vi "3458A Initiate Digitizing Process.vi"(8 "error in":errorcluster, 9 "Is first multiplex cycle? (True)":bool, 11 "session in":T1={"channels"=[], "sync unit"={"VISA"="", "type"=enum."Picotest U6200A"}, "awg unit"={"type"=enum."Agilent 331xxA to 332xxA", "VISA"="", "enable 10MHz ref"=FALSE, "cmi ckd2"={"VISA"="", "clock source"=enum."Auto", "manual ref clk"=FALSE, "ref clock [Hz]"=0.0, "div mode"=enum."Set divisor directly"}, "cmi sync v3"={"VISA"="", "baud rate [bd/s]"=115200, "source"=enum."Auto", "hv range"=enum."1kV", "fsrc is fixed"=FALSE, "fsrc [Hz]"=10000000.0, "freq integ [s]"=1.0, "freq filter"=5, "trig level"=enum."TTL 5V", "chn1 mode"=enum."Source divider", "chn1 level"=enum."Positive 5V", "chn2 mode"=enum."Source divider", "chn2 level"=enum."Positive 5V", "chn2 div"=1, "chn3 mode"=enum."Chn 1 Active", "chn3 level"=enum."Positive 5V", "chn1 div entry"=enum."Calculate nearest divisor from measured fx", "chn1 dev limit [%]"=1.0, "chn1 check dev"=FALSE}, "trigger"={"source"=enum."Immediate", "slope"=enum."POS", "coupling"=enum."DC", "level [V]"=0.0, "hysteresis [V]"=0.0, "pre-trigger [%]"=0.0}, "HMF2500 cfg"={"Baud Rate"=9600, "Parity"=0, "Data Bits"=8, "Flow Control"=4}}, "sync mode"=enum."MASTER-SLAVE, MASTER clocked by TIMER", "streaming mode"=FALSE, "idn mode"=enum."Auto", "sampling mode"=enum."DCV", "sample memory [B]"=0, "proc setup"={"channel id"=0, "packet size [smpl]"=0, "current timeout [s]"=0.0, "blk2blk timeout [s]"=0.0, "event time"=timestamp(0 s since 1904-01-01), "stop notifier"=refnum, "data queues"=[], "proc refs"=[], "bus semaphore"=refnum}, "sample size [B]"=0, "sample count"=0, "aux data"={"channel id"=0, "valid?"=[], "gain [V]"=[], "timestamp [s]"=[], "Ts [s]"=0.0, "abs timestamp"=timestamp(0 s since 1904-01-01), "t [deg C]"=[], "multiplex timestamp [s]"=-1.0, "only multiplex?"=FALSE, "multiplex smpl offset"=0, "overflow?"=FALSE}, "ranges [V]"=[], "aperture [s]"=0.0, "LEVEL trigger"={"edge"=enum."POS", "level [V]"=0.0, "coupling"=enum."DC"}, "trigger mode"=enum."AUTO", "measure temp.?"=FALSE, "disp mesages"=[], "shared bus?"=FALSE, "disable display?"=FALSE, "aper mode"=enum."Manual", "aper rules"=[], "multiplex"={"cycles"=0, "delay [s]"=0.0, "enabled"=FALSE, "overhead [s]"=1.0, "tot smpls"=0, "sub-rec"=0, "overhead [%]"=0.0, "emulated"=FALSE}, "F8588 lpf"=enum."Off", "F8588 pll"=enum."Off", "F8588 couple"=enum."DC, auto", "fs"={"freq mode"=enum."fs or Ts", "fs [Hz]"=0.0, "fref [Hz]"=0.0, "mul"=0.0, "div"=0.0}, "fs mode"=enum."fs or Ts", "init timestamp"=timestamp(0 s since 1904-01-01), "last report timestamp"=timestamp(0 s since 1904-01-01)} {"awg unit"."HMF2500 cfg"."Flow Control" items=["None", "XON/XOFF", "RTS/CTS", "XON/XOFF & RTS/CTS", "DTR/DSR", "XON/XOFF & DTR/DSR"]; "awg unit"."HMF2500 cfg"."Data Bits" items=["7"=7, "8"=8]; "awg unit"."HMF2500 cfg"."Parity" items=["None", "Odd", "Even", "Mark", "Space"]; "awg unit"."HMF2500 cfg"."Baud Rate" items=["300"=300, "600"=600, "1200"=1200, "2400"=2400, "4800"=4800, "9600"=9600, "19200"=19200]; "awg unit"."cmi sync v3"."chn2 div" min=1 max=100000000 step=1; "awg unit"."cmi sync v3"."fsrc [Hz]" format="%_8p"; "channels"."Range [Vpk]" min=0.0}) -> (0 "error out":errorcluster, 2 "initiation timestamp":timestamp, 3 "session out":T1={"channels"=[], "sync unit"={"VISA"="", "type"=enum."Picotest U6200A"}, "awg unit"={"type"=enum."Agilent 331xxA to 332xxA", "VISA"="", "enable 10MHz ref"=FALSE, "cmi ckd2"={"VISA"="", "clock source"=enum."Auto", "manual ref clk"=FALSE, "ref clock [Hz]"=0.0, "div mode"=enum."Set divisor directly"}, "cmi sync v3"={"VISA"="", "baud rate [bd/s]"=115200, "source"=enum."Auto", "hv range"=enum."1kV", "fsrc is fixed"=FALSE, "fsrc [Hz]"=10000000.0, "freq integ [s]"=1.0, "freq filter"=5, "trig level"=enum."TTL 5V", "chn1 mode"=enum."Source divider", "chn1 level"=enum."Positive 5V", "chn2 mode"=enum."Source divider", "chn2 level"=enum."Positive 5V", "chn2 div"=1, "chn3 mode"=enum."Chn 1 Active", "chn3 level"=enum."Positive 5V", "chn1 div entry"=enum."Calculate nearest divisor from measured fx", "chn1 dev limit [%]"=1.0, "chn1 check dev"=FALSE}, "trigger"={"source"=enum."Immediate", "slope"=enum."POS", "coupling"=enum."DC", "level [V]"=0.0, "hysteresis [V]"=0.0, "pre-trigger [%]"=0.0}, "HMF2500 cfg"={"Baud Rate"=9600, "Parity"=0, "Data Bits"=8, "Flow Control"=4}}, "sync mode"=enum."MASTER-SLAVE, MASTER clocked by TIMER", "streaming mode"=FALSE, "idn mode"=enum."Auto", "sampling mode"=enum."DCV", "sample memory [B]"=0, "proc setup"={"channel id"=0, "packet size [smpl]"=0, "current timeout [s]"=0.0, "blk2blk timeout [s]"=0.0, "event time"=timestamp(0 s since 1904-01-01), "stop notifier"=refnum, "data queues"=[], "proc refs"=[], "bus semaphore"=refnum}, "sample size [B]"=0, "sample count"=0, "aux data"={"channel id"=0, "valid?"=[], "gain [V]"=[], "timestamp [s]"=[], "Ts [s]"=0.0, "abs timestamp"=timestamp(0 s since 1904-01-01), "t [deg C]"=[], "multiplex timestamp [s]"=-1.0, "only multiplex?"=FALSE, "multiplex smpl offset"=0, "overflow?"=FALSE}, "ranges [V]"=[], "aperture [s]"=0.0, "LEVEL trigger"={"edge"=enum."POS", "level [V]"=0.0, "coupling"=enum."DC"}, "trigger mode"=enum."AUTO", "measure temp.?"=FALSE, "disp mesages"=[], "shared bus?"=FALSE, "disable display?"=FALSE, "aper mode"=enum."Manual", "aper rules"=[], "multiplex"={"cycles"=0, "delay [s]"=0.0, "enabled"=FALSE, "overhead [s]"=1.0, "tot smpls"=0, "sub-rec"=0, "overhead [%]"=0.0, "emulated"=FALSE}, "F8588 lpf"=enum."Off", "F8588 pll"=enum."Off", "F8588 couple"=enum."DC, auto", "fs"={"freq mode"=enum."fs or Ts", "fs [Hz]"=0.0, "fref [Hz]"=0.0, "mul"=0.0, "div"=0.0}, "fs mode"=enum."fs or Ts", "init timestamp"=timestamp(0 s since 1904-01-01), "last report timestamp"=timestamp(0 s since 1904-01-01)} {"awg unit"."HMF2500 cfg"."Flow Control" items=["None", "XON/XOFF", "RTS/CTS", "XON/XOFF & RTS/CTS", "DTR/DSR", "XON/XOFF & DTR/DSR"]; "awg unit"."HMF2500 cfg"."Data Bits" items=["7"=7, "8"=8]; "awg unit"."HMF2500 cfg"."Parity" items=["None", "Odd", "Even", "Mark", "Space"]; "awg unit"."HMF2500 cfg"."Baud Rate" items=["300"=300, "600"=600, "1200"=1200, "2400"=2400, "4800"=4800, "9600"=9600, "19200"=19200]; "awg unit"."cmi sync v3"."chn2 div" min=1 max=100000000 step=1; "awg unit"."cmi sync v3"."fsrc [Hz]" format="%_8p"; "channels"."Range [Vpk]" min=0.0})   [LabVIEW 2020, in "3458A Virtual Digitizer.lvlib"]
doc: "Initiates acquisition for both single shot and streaming modes. It creates data queues and starts digitizing processes, one for each channel. If succeds the process immediatelly starts digitizing (after trigger event occures) and starts filling the queues with data. So this VI must be immediatelly followed by fetch loop that takes out data from the queue! This may be called repeatedely without calling 'Setup' function if multiple records are required with identical configuration.\n\nFor time multiplexing mode set 'Time multiplex mode = True'. When 'Is first multiplex cycle = True', it will initiate record of maximum possible size. For next multiplexing cycles set 'Is first multiplex cycle = False' which will just record timestamp. The timestamps from particular calls of this VI will be later used to split the long record to particular multiplexing sequence chunks."
uses:
  3458A Virtual Digitizer.lvlib
  3458A Digitizer Session.ctl
  3458A Virtual Channel Config.ctl
  Counter/Counter Session.ctl
  Counter/Counter Type.ctl
  AWG/AWG Session.ctl
  AWG/AWG Type.ctl
  AWG/CMI Clock Divider v2/CMI ckd2 Session.ctl
  AWG/CMI Clock Divider v2/CMI ckd2 Source Mode.ctl
  AWG/CMI Clock Divider v2/CMI ckd2 Divisor Mode.ctl
  AWG/CMI Sync V3/CMI Sync V3 session.ctl
  AWG/CMI Sync V3/Configure/CMI Sync V3 Reference Clock Source.ctl
  AWG/CMI Sync V3/Configure/CMI Sync V3 HV input Range.ctl
  AWG/CMI Sync V3/Configure/CMI Sync V3 Trigger Input Level.ctl
  AWG/CMI Sync V3/Configure/CMI Sync V3 Channel 1 Mode.ctl
  AWG/CMI Sync V3/Configure/CMI Sync V3 Channel Output Levels.ctl
  AWG/CMI Sync V3/Configure/CMI Sync V3 Channel 2 Mode.ctl
  AWG/CMI Sync V3/Configure/CMI Sync V3 Channel 3 Mode.ctl
  AWG/CMI Sync V3/Configure/CMI Sync V3 Channel 1 Divisor Entry Mode.ctl
  adc/ADC Trig Config.ctl
  adc/ADC Trig Mode Source.ctl
  adc/ADC Trig Slope.ctl
  adc/ADC Trig Coupling.ctl
  AWG/RaS HMF2500/HMF2500 Config.ctl
  3458A Sync Mode.ctl
  3458A Idn Mode.ctl
  3458A Digitizing Low Levels/Configure/Sampling Mode.ctl
  3458A Digitizing Process Options.ctl
  3458A Data Packet.ctl
  3458A Aux Record Data.ctl
  3458A Digitizing Low Levels/Configure/Level Setup.ctl
  3458A Digitizing Low Levels/Configure/First Sample Trigger.ctl
  3458A Aperture Selection Mode.ctl
  3458A Multiplexing Config.ctl
  Fluke 8588A/F8588A Low Pass Filter.ctl
  Fluke 8588A/F8588A Phase Lock.ctl
  Fluke 8588A/F8588A Coupling.ctl
  3458A Sampling Rate.ctl
  AWG/AWG Clock Setup Mode.ctl
  3458A Sample Rate Mode.ctl
  AWG/AWG.lvlib
  Counter/Counter.lvlib
  3458A Digitizing Low Levels/3458A Digitizing Low Levels.lvlib
  AWG/CMI Sync V3/CMI Sync Unit V3.lvlib
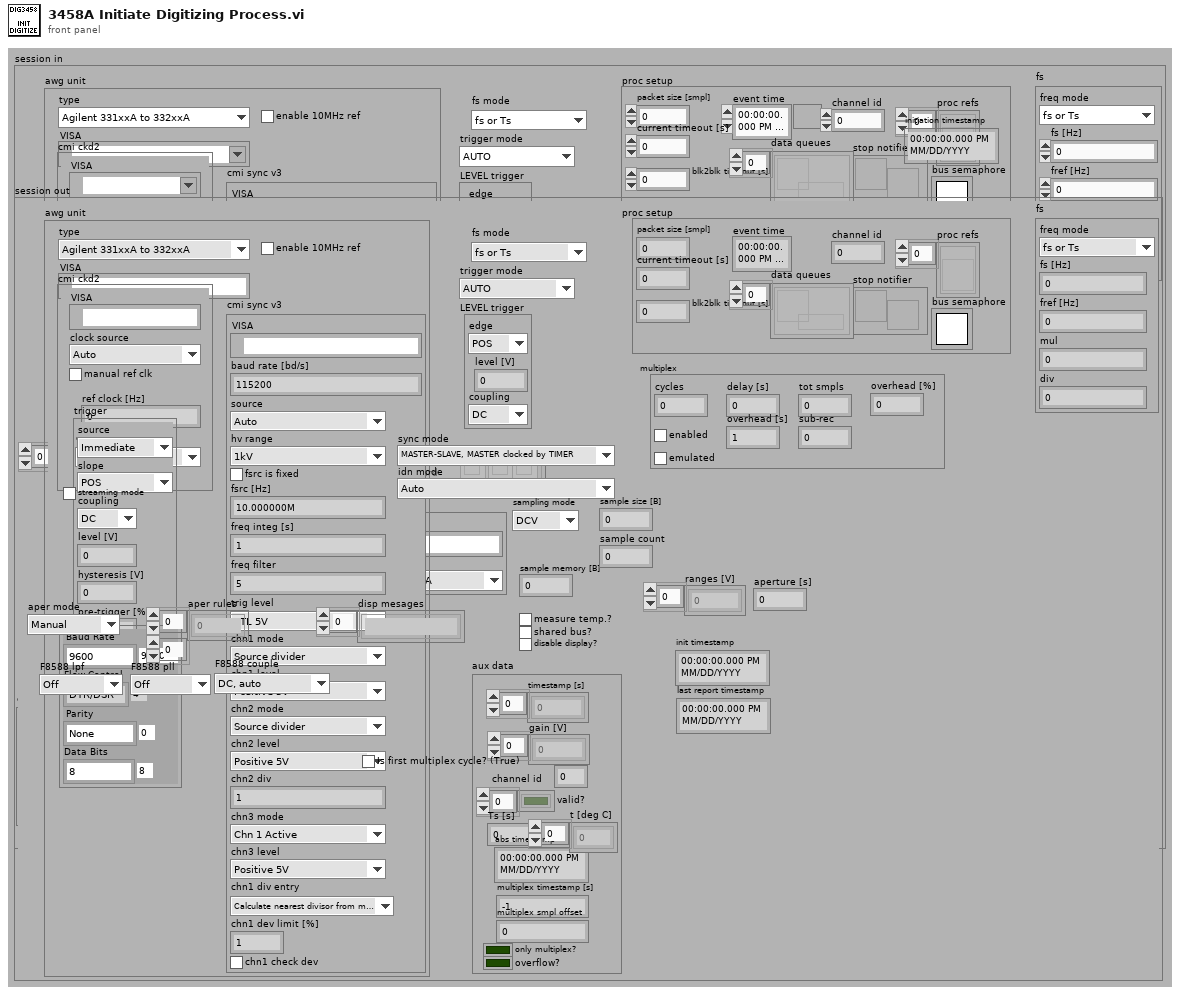
[diagram p1: front panel]
types:
  T1 = typedef "3458A Virtual Digitizer.lvlib/3458A Digitizer Session.ctl" = cluster{"channels":T2[], "sync unit":T3, "awg unit":T5, "sync mode":T24, "streaming mode":bool, "idn mode":T25, "sampling mode":T26, "sample memory [B]":i32, "proc setup":T27, "sample size [B]":i32, "sample count":i32, "aux data":T29, "ranges [V]":dbl[], "aperture [s]":dbl, "LEVEL trigger":T30, "trigger mode":T31, "measure temp.?":bool, "disp mesages":string[], "shared bus?":bool, "disable display?":bool, "aper mode":T32, "aper rules":dbl[][], "multiplex":T33, "F8588 lpf":T34, "F8588 pll":T35, "F8588 couple":T36, "fs":T37, "fs mode":T39, "init timestamp":timestamp, "last report timestamp":timestamp}
  T2 = typedef "3458A Virtual Digitizer.lvlib/3458A Virtual Channel Config.ctl" = cluster{"VISA":refnum<visa-resource-name>, "Range [Vpk]":dbl, "btn clr":bool, "btn up":bool, "btn down":bool, "F8588":bool, "F8588 guard":bool}
  T3 = typedef "Counter.lvlib/Counter Session.ctl" = cluster{"VISA":refnum<visa-resource-name>, "type":T4}
  T4 = typedef "Counter.lvlib/Counter Type.ctl" = enum16{"Picotest U6200A", "dummy"}
  T5 = typedef "AWG.lvlib/AWG Session.ctl" = cluster{"type":T6, "VISA":refnum<visa-resource-name>, "enable 10MHz ref":bool, "cmi ckd2":T7, "cmi sync v3":T10, "trigger":T19, "HMF2500 cfg":T23}
  T6 = typedef "AWG.lvlib/AWG Type.ctl" = enum16{"Agilent 331xxA to 332xxA", "Agilent 335xxA to 336xxA", "Tektronix AFG3101C", "R&S HMF25xx", "CMI Clock Divider v2", "CMI Sync Unit V3", "dummy"}
  T7 = typedef "AWG.lvlib/CMI ckd2 Session.ctl" = cluster{"VISA":refnum<visa-resource-name>, "clock source":T8, "manual ref clk":bool, "ref clock [Hz]":dbl, "div mode":T9}
  T8 = typedef "AWG.lvlib/CMI ckd2 Source Mode.ctl" = enum16{"Auto", "LF clock", "HF clock", "Internal"}
  T9 = typedef "AWG.lvlib/CMI ckd2 Divisor Mode.ctl" = enum16{"Set divisor directly", "Set divisor by frequency"}
  T10 = typedef "AWG.lvlib/CMI Sync Unit V3.lvlib/CMI Sync V3 session.ctl" = cluster{"VISA":refnum<visa-resource-name>, "baud rate [bd/s]":i32, "source":T11, "hv range":T12, "fsrc is fixed":bool, "fsrc [Hz]":dbl, "freq integ [s]":dbl, "freq filter":i32, "trig level":T13, "chn1 mode":T14, "chn1 level":T15, "chn2 mode":T16, "chn2 level":T15, "chn2 div":i32, "chn3 mode":T17, "chn3 level":T15, "chn1 div entry":T18, "chn1 dev limit [%]":dbl, "chn1 check dev":bool}
  T11 = typedef "AWG.lvlib/CMI Sync Unit V3.lvlib/CMI Sync V3 Reference Clock Source.ctl" = enum16{"Auto", "Internal", "Logic", "Sine", "HV"}
  T12 = typedef "AWG.lvlib/CMI Sync Unit V3.lvlib/CMI Sync V3 HV input Range.ctl" = enum16{"10V", "60V", "250V", "1kV"}
  T13 = typedef "AWG.lvlib/CMI Sync Unit V3.lvlib/CMI Sync V3 Trigger Input Level.ctl" = enum16{"LVCMOS 3V3", "TTL 5V"}
  T14 = typedef "AWG.lvlib/CMI Sync Unit V3.lvlib/CMI Sync V3 Channel 1 Mode.ctl" = enum16{"Source divider", "DDS absolute", "DDS ratio", "DDS ratio M/N"}
  T15 = typedef "AWG.lvlib/CMI Sync Unit V3.lvlib/CMI Sync V3 Channel Output Levels.ctl" = enum16{"Positive 3V3", "Negative 3V3", "Positive 5V", "Negative 5V"}
  T16 = typedef "AWG.lvlib/CMI Sync Unit V3.lvlib/CMI Sync V3 Channel 2 Mode.ctl" = enum16{"Source divider", "Chn 1 divide"}
  T17 = typedef "AWG.lvlib/CMI Sync Unit V3.lvlib/CMI Sync V3 Channel 3 Mode.ctl" = enum16{"Chn 1 Active", "Chn 2 Active", "Chn 1 Trigger", "Chn 2 Trigger", "Gate", "PPS", "10MHz"}
  T18 = typedef "AWG.lvlib/CMI Sync Unit V3.lvlib/CMI Sync V3 Channel 1 Divisor Entry Mode.ctl" = enum16{"Set divisor directly", "Calculate nearest divisor from measured fx"}
  T19 = typedef "ADC Trig Config.ctl" = cluster{"source":T20, "slope":T21, "coupling":T22, "level [V]":dbl, "hysteresis [V]":dbl, "pre-trigger [%]":dbl}
  T20 = typedef "ADC Trig Mode Source.ctl" = enum16{"Immediate", "External", "Level"}
  T21 = typedef "ADC Trig Slope.ctl" = enum16{"POS", "NEG"}
  T22 = typedef "ADC Trig Coupling.ctl" = enum16{"DC", "AC"}
  T23 = typedef "AWG.lvlib/HMF2500 Config.ctl" = cluster{"Baud Rate":u32, "Parity":u16, "Data Bits":u16, "Flow Control":u16}
  T24 = typedef "3458A Virtual Digitizer.lvlib/3458A Sync Mode.ctl" = enum16{"MASTER-SLAVE, MASTER clocked by TIMER", "MASTER-SLAVE, MASTER clocked by AWG", "ALL clocked by AWG", "MASTER-SLAVE, ALL clocked by TIMER", "ALL clocked by AWG with DFLL"}
  T25 = typedef "3458A Virtual Digitizer.lvlib/3458A Idn Mode.ctl" = enum16{"Auto", "Sequential (chn A, chn B, ...)", "From calibration string"}
  T26 = typedef "3458A Virtual Digitizer.lvlib/3458A Digitizing Low Levels.lvlib/Sampling Mode.ctl" = enum16{"DCV", "DSDC", "DSAC"}
  T27 = typedef "3458A Virtual Digitizer.lvlib/3458A Digitizing Process Options.ctl" = cluster{"channel id":i32, "packet size [smpl]":i32, "current timeout [s]":dbl, "blk2blk timeout [s]":dbl, "event time":timestamp, "stop notifier":refnum<notifier>, "data queues":refnum<queue>[], "proc refs":refnum<vi>[], "bus semaphore":T28}
  T28 = typedef "Semaphore RefNum" = refnum<k1>
  T29 = typedef "3458A Virtual Digitizer.lvlib/3458A Aux Record Data.ctl" = cluster{"channel id":i32, "valid?":bool[], "gain [V]":dbl[], "timestamp [s]":dbl[], "Ts [s]":dbl, "abs timestamp":timestamp, "t [deg C]":dbl[], "multiplex timestamp [s]":dbl, "only multiplex?":bool, "multiplex smpl offset":i64, "overflow?":bool}
  T30 = typedef "3458A Virtual Digitizer.lvlib/3458A Digitizing Low Levels.lvlib/Level Setup.ctl" = cluster{"edge":enum16{"POS", "NEG"}, "level [V]":dbl, "coupling":enum16{"DC", "AC"}}
  T31 = typedef "3458A Virtual Digitizer.lvlib/3458A Digitizing Low Levels.lvlib/First Sample Trigger.ctl" = enum16{"AUTO", "EXT", "SYN", "SGL", "HOLD", "LEVEL"}
  T32 = typedef "3458A Virtual Digitizer.lvlib/3458A Aperture Selection Mode.ctl" = enum16{"Manual", "Maximum", "Table"}
  T33 = typedef "3458A Virtual Digitizer.lvlib/3458A Multiplexing Config.ctl" = cluster{"cycles":i32, "delay [s]":dbl, "enabled":bool, "overhead [s]":dbl, "tot smpls":i64, "sub-rec":i32, "overhead [%]":dbl, "emulated":bool}
  T34 = typedef "F8588A Low Pass Filter.ctl" = enum16{"Off", "100 kHz", "3 MHz"}
  T35 = typedef "F8588A Phase Lock.ctl" = enum16{"Off", "1 MHz", "10 MHz"}
  T36 = typedef "F8588A Coupling.ctl" = enum16{"AC, 1 MOhm", "AC, 10 MOhm", "DC, 1 MOhm", "DC, 10 MOhm", "DC, auto"}
  T37 = typedef "3458A Virtual Digitizer.lvlib/3458A Sampling Rate.ctl" = cluster{"freq mode":T38, "fs [Hz]":dbl, "fref [Hz]":dbl, "mul":dbl, "div":dbl}
  T38 = typedef "AWG.lvlib/AWG Clock Setup Mode.ctl" = enum16{"fs or Ts", "fs or Ts with fref", "fref/N", "fref*M/N", "fref*Ratio"}
  T39 = typedef "3458A Sample Rate Mode.ctl" = enum16{"fs or Ts", "fs*M/N"}
  T40 = typedef "3458A Virtual Digitizer.lvlib/3458A Data Packet.ctl" = cluster{"data":i32[][], "offset [smpl]":i32, "count [smpl]":i32, "all done?":bool, "sampling?":bool, "queue buffer [%]":dbl, "valid?":bool, "overflow?":bool, "estimate info?":bool}
  T41 = typedef "3458A Virtual Digitizer.lvlib/3458A Capabilities.ctl" = cluster{"max samples count":i64, "max fs [Hz]":ext, "min fs [Hz]":ext, "Ts step [s]":ext, "max Ts [s]":ext, "min Ts [s]":ext, "allows streaming?":bool, "streaming on?":bool, "has level trig?":bool, "has ext trig?":bool, "min aperture [s]":dbl, "max aperture [s]":dbl, "has aperture?":bool, "channels count":i32, "has temp.?":bool, "fs step [Hz]":ext, "const fs step?":bool, "no aper info":string, "has timestamps?":bool, "freq mode":T38, "auto aperture?":bool, "can select fs mode?":bool}
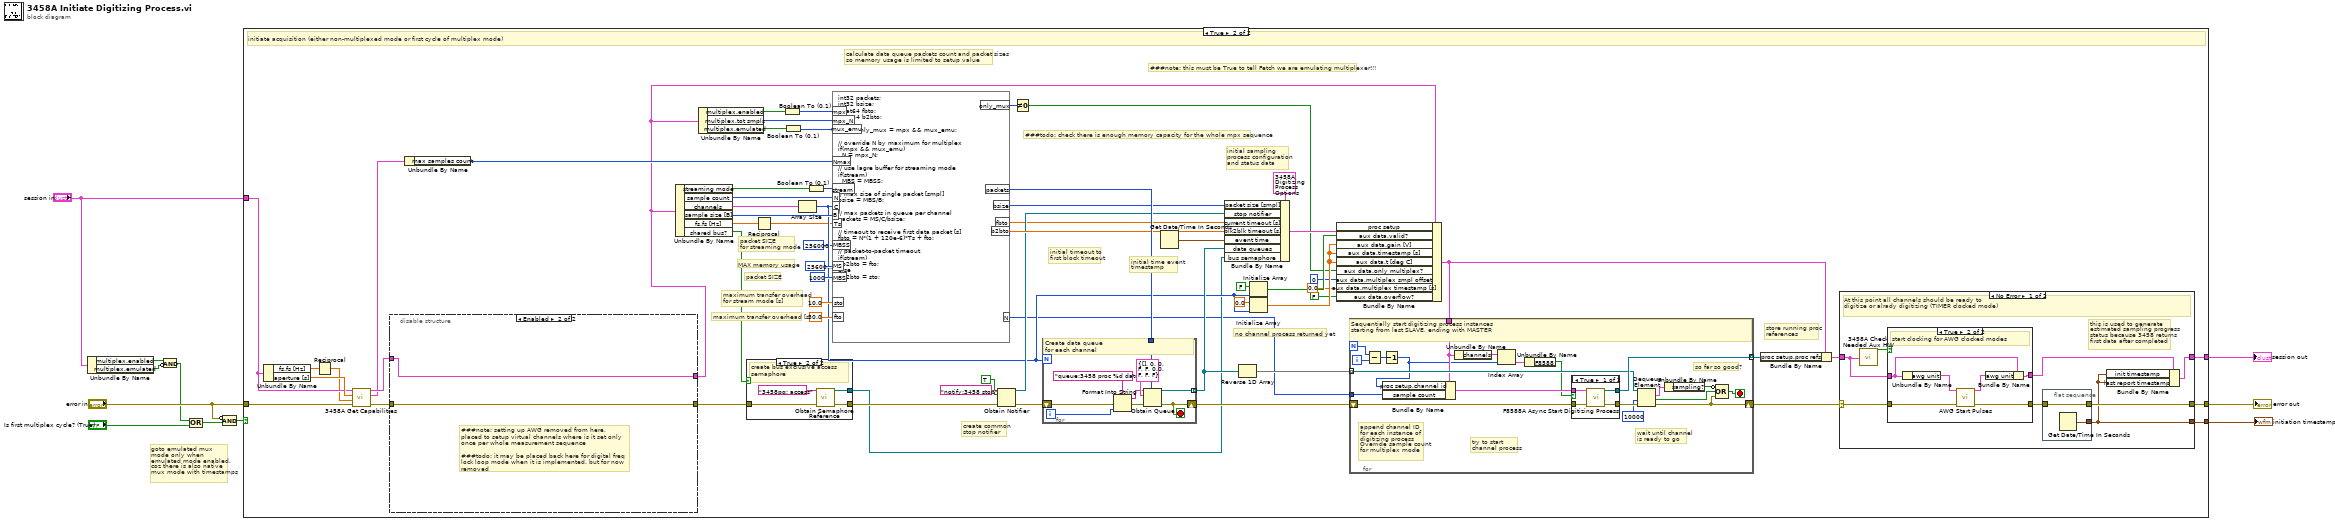
[diagram p0: block diagram]
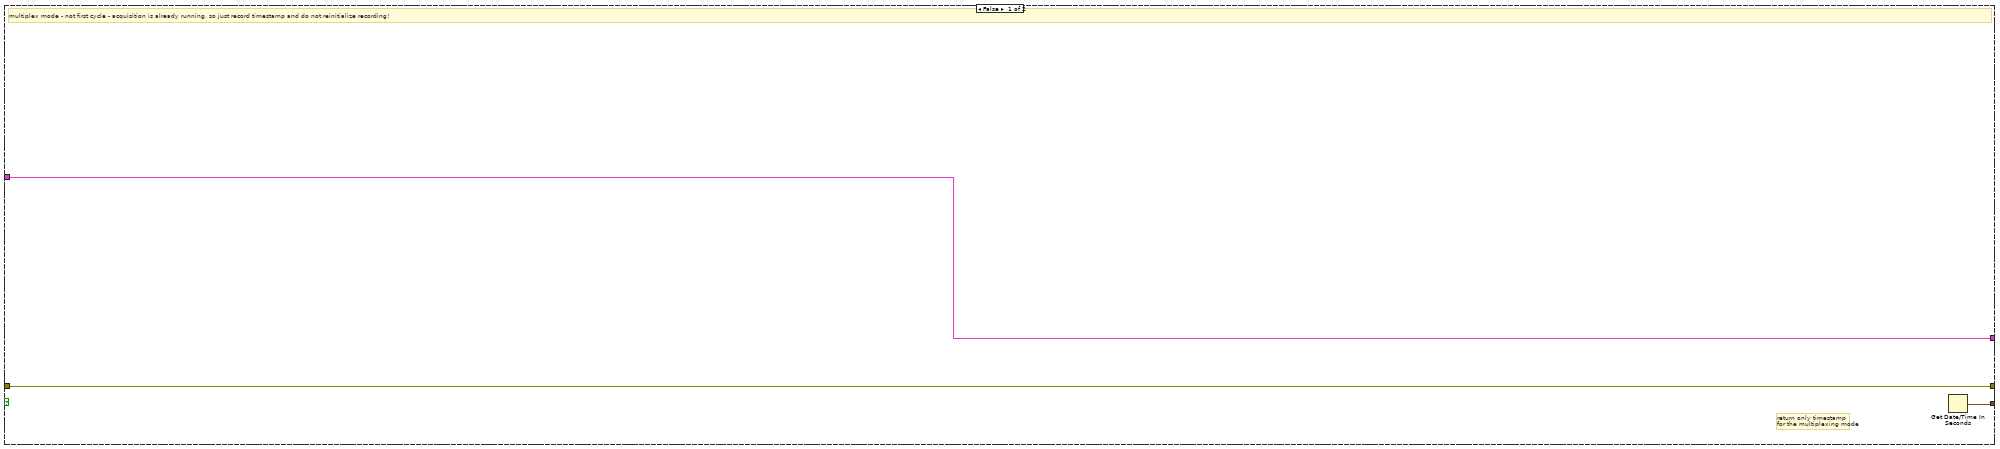
[diagram p2: hidden frame]
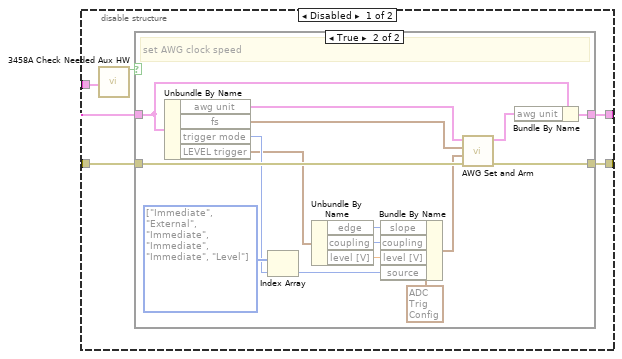
[diagram p3: hidden frame]
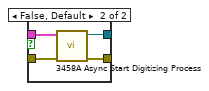
[diagram p8: hidden frame]
diagram:
  # "goto emulated mux\nmode only when \nemulated mode enabled,\ncoz there is also native\nmux mode with timestamps"
  n1 = Unbundle By Name("session in") -> ("multiplex.enabled"=w5:bool, "multiplex.emulated"=w4:bool)
  n2 = Compound Arithmetic op=AND(w5, invert w4) -> (w2:bool)
  n3 = Compound Arithmetic op=OR(w2, "Is first multiplex cycle? (True)") -> (w3:bool)
  n4 = Compound Arithmetic op=AND(invert "error in", w3) -> (w9:bool)
  n5 = case shown="True" w9 {
    tunnel: [w13 w53] -> w11
    tunnel: "session in" -> [w14 w22]
    tunnel: [w14 w52] -> w10
    tunnel: "error in" -> [w13 w37]
    tunnel: [w12 w30] -> w7
    frame False {
      # "return only timestamp\nfor the multiplexing mode"
      # "multiplex mode - not first cycle - acquisition is already running, so just record timestamp and do not reinitialize recording!"
      n6 = Get Date/Time In Seconds() -> (seconds since 1Jan1904=w12:timestamp)
    }
    frame True {
      # "###note: this must be True to tell Fetch we are emulating multiplexer!!!"
      # "###todo: check there is enough memory capacity for the whole mpx sequence"
      # "packet SIZE\nfor streaming mode"
      # "no channel process returned yet"
      # "initial time event\ntimestamp"
      # "maximum transfer overhead\nfor stream mode [s]"
      # "store running proc\nreferences"
      # "create common\nstop notifier"
      # "initial timeout to\nfirst block timeout"
      # "maximum transfer overhead [s]"
      # "initial sampling\nprocess configuration\nand status data"
      # "calculate data queue packets count and packet sizes\nso memory usage is limited to setup value"
      # "packet SIZE"
      # "MAX memory usage"
      # "initiate acquisition (either non-multiplexed mode or first cycle of multiplex mode)"
      n7 = Unbundle By Name(w22) -> ("fs.fs [Hz]"=w34:dbl, "aperture [s]"=w33:dbl)
      n8 = Reciprocal(x=w34) -> (1/x=w16:dbl)
      n9 = call "3458A Get Capabilities.vi"("error in"=w37, "Ts [s]"=w16, "aperture [s]"=w33, "digitizer session in"=w22) -> ("error out"=w36:errorcluster, "capabilities"=w27:T41, "digitizer session out"=w35:T1)  [unwired: 5 in]
      n10 = disable-structure shown="Enabled" {
        disable-tunnel: [w82 w102] -> w38
        disable-tunnel: w36 -> [w80 w102]
        disable-tunnel: w35 -> [w79 w101]
        disable-tunnel: [w78 w101] -> w26
        frame Disabled {
          n11 = call "3458A Check Needed Aux HW.vi"("digitizer session"=w79) -> ("uses AWG clocking?"=w81:bool)  [unwired: 13 in, 5 out]
          n12 = case shown="True" w81 {
            tunnel: w80 -> [w83 w100]
            tunnel: w79 -> [w84 w97]
            tunnel: [w83 w96] -> w82
            tunnel: [w84 w95] -> w78
            frame False {
              # "do nothing for TIMER clocked modes"
            }
            frame True {
              w91 = T20[] [enum."Immediate", enum."External", enum."Immediate", enum."Immediate", enum."Immediate", enum."Level"] items=["Immediate", "External", "Level"]
              # "set AWG clock speed"
              n13 = Unbundle By Name(w97) -> ("awg unit"=w99:T5, "fs"=w94:T37, "trigger mode"=w90:T31, "LEVEL trigger"=w88:T30)
              n14 = Index Array(array=w91, index=w90) -> (element=w89:T20)
              n15 = Unbundle By Name(w88) -> ("edge"=w85:enum16{"POS", "NEG"}, "coupling"=w86:enum16{"DC", "AC"}, "level [V]"=w87:dbl)
              n16 = Bundle By Name(cluster=T19 {"source"=enum."Immediate", "slope"=enum."POS", "coupling"=enum."DC", "level [V]"=0.0, "hysteresis [V]"=0.0, "pre-trigger [%]"=0.0} ("trigger"), "slope"=w85, "coupling"=w86, "level [V]"=w87, "source"=w89) -> (w92:T19)
              n17 = call "AWG Set and Arm.vi"("error in (no error)"=w100, "trigger"=w92, "sampling rate"=w94, "awg session in"=w99) -> ("error out"=w96:errorcluster, "awg session out"=w98:T5)  [unwired: 6 in]
              n18 = Bundle By Name(cluster=w97, "awg unit"=w98) -> (w95:T1)
            }
          }
        }
        frame Enabled {
          # "###note: setting up AWG removed from here,\nplaced to setup virtual channels where is it set only\nonce per whole measurement sequence\n\n###todo: it may be placed back here for digital freq\nlock loop mode when it is implemented, but for now removed"
        }
      }
      n19 = Unbundle By Name(w27) -> ("max samples count"=w32:i64)
      n20 = Unbundle By Name(w26) -> ("streaming mode"=w76:bool, "sample count"=w74:i32, "channels"=w73:T2[], "sample size [B]"=w51:i32, "fs.fs [Hz]"=w50:dbl, "shared bus?"=w41:bool)
      n21 = Unbundle By Name(w26) -> ("multiplex.enabled"=w18:bool, "multiplex.tot smpls"=w24:i64, "multiplex.emulated"=w21:bool)
      n22 = case shown="True" w41 {
        tunnel: w38 -> [w103 w107]
        tunnel: [w103 w106] -> w42
        tunnel: [_ w104] -> w40
        frame False {
        }
        frame True {
          # "create bus exclusive access\nsemaphore"
          n23 = call <vilib>:"Obtain Semaphore Reference.vi"("error in (no error)"=w107, "name (unnamed)"="3458pq: access") -> ("error out"=w106:errorcluster, "semaphore"=w104:T28)  [unwired: 3 in, 1 out]
        }
      }
      n24 = Reciprocal(x=w50) -> (1/x=w15:dbl)
      n25 = Boolean To (0,1)(Boolean=w18) -> (0, 1=w25:i16)
      n26 = Boolean To (0,1)(Boolean=w21) -> (0, 1=w20:i16)
      n27 = Array Size(array=w73) -> (size(s)=w44:i32)
      n28 = Boolean To (0,1)(Boolean=w76) -> (0, 1=w75:i16)
      n29 = formula code="int32 packets;\nint32 bsize;\nfloat64 fbto;\nfloat64 b2bto;\n\nint32 only_mux = mpx && mux_emu;\n\n// override N by maximum for multiplex\nif(mpx && mux_emu)\n  N = mpx_N;\n\n// use lagre buffer for streaming mode\nif(stream)\n  MBS = MBSS;\n\n// max size of single packet [smpl]\nbsize = MBS/B;\n\n// max packets in queue per channel\npackets = MS/C/bsize;\n\n// timeout to receive first data packet [s]\nfbto = N*(1 + 120e-6)*Ts + fto;\n\n// packet-to-packet timeout\nif(stream)\n  b2bto = fto;\nelse\n  b2bto = sto;"("stream"=w75, "N"=w74, "C"=w44, "MS"=256000000 ("y"), "MBS"=1000 ("y"), "Ts"=w15, "fto"=30.0 ("input variable"), "B"=w51, "sto"=10.0 ("input variable"), "MBSS"=256000 ("y"), "Nmax"=w32, "mpx"=w25, "mpx_N"=w24, "mux_emu"=w20) -> ("packets"=w70:i32, "bsize"=w69:i32, "fbto"=w48:dbl, "b2bto"=w65:dbl, "N"=w31:i32, "only_mux"=w19:i32)
      n30 = Obtain Notifier(name (unnamed)="notify:3458 stop", notification data type=TRUE, error in (no error)=w42) -> (notifier out=w61:refnum<notifier>, error out=w63:errorcluster)  [unwired: 1 in, 1 out]
      n31 = Not Equal To 0?(x=w19) -> (x != 0?=w17:bool)
      n32 = for {
        N: w44 -> [_]
        tunnel: w70 -> [w164]
        shift-right: [w156] -> w68
        shift-left: w63 -> [w161]
        tunnel: [w162] -> w58 mode=indexing
        i -> [w157]
        stop <- w156 stop-if-true
        # "Create data queue\nfor each channel"
        n33 = Format Into String(format string="queue:3458 proc %d data" ("name (unnamed)"), error in=w161, w157) -> (resulting string=w159:string, error out=w160:errorcluster)  [unwired: 1 in]
        n34 = Obtain Queue(max queue size (-1, unlimited)=w164, name (unnamed)=w159, element data type=T40 {"data"=[], "offset [smpl]"=0, "count [smpl]"=0, "all done?"=FALSE, "sampling?"=FALSE, "queue buffer [%]"=0.0, "valid?"=FALSE, "overflow?"=FALSE, "estimate info?"=FALSE} ("niScope packet"), error in (no error)=w160) -> (queue out=w162:refnum<queue>, error out=w156:errorcluster)  [unwired: 1 in, 1 out]
      }
      n35 = Get Date/Time In Seconds() -> (seconds since 1Jan1904=w66:timestamp)
      n36 = Bundle By Name(cluster=T27 {"channel id"=0, "packet size [smpl]"=0, "current timeout [s]"=0.0, "blk2blk timeout [s]"=0.0, "event time"=timestamp(0 s since 1904-01-01), "stop notifier"=refnum, "data queues"=[], "proc refs"=[], "bus semaphore"=refnum} ("setup"), "packet size [smpl]"=w69, "stop notifier"=w61, "current timeout [s]"=w48, "blk2blk timeout [s]"=w65, "event time"=w66, "data queues"=w58, "bus semaphore"=w40) -> (w60:T27)
      n37 = Reverse 1D Array(array=w58) -> (reversed array=w59:refnum<queue>[])
      n38 = Initialize Array(FALSE, w44) -> (w47:bool[])
      n39 = Initialize Array(0.0, w44) -> (w43:dbl[])
      n40 = Bundle By Name(cluster=w26, "proc setup"=w60, "aux data.valid?"=w47, "aux data.gain [V]"=w43, "aux data.timestamp [s]"=w43, "aux data.t [deg C]"=w43, "aux data.only multiplex?"=w17, "aux data.multiplex smpl offset"=i64 0, "aux data.multiplex timestamp [s]"=0.0, "aux data.overflow?"=FALSE) -> (w56:T1)
      n41 = for {
        N -> [w141]
        tunnel: [w146] -> w55 mode=indexing
        tunnel: w56 -> [w132]
        tunnel: w59 -> [w144] mode=indexing
        shift-right: [w138] -> w57
        shift-left: w68 -> [w147]
        tunnel: w31 -> [w133]
        i -> [w140]
        stop <- w136 stop-if-true
        # "so far so good?"
        # "wait until channel\nis ready to go"
        # "try to start\nchannel process"
        # "append channel ID\nfor each instance of\ndigitizing process\nOverride sample count\nfor multiplex mode"
        # "Sequentially start digitizing process instances\nstarting from last SLAVE, ending with MASTER"
        n42 = Subtract(x=w141, y=w140) -> (x-y=w139:i32)
        n43 = Decrement(x=w139) -> (x-1=w130:i32)
        n44 = Bundle By Name(cluster=w132, "proc setup.channel id"=w130, "sample count"=w133) -> (w142:T1)
        n45 = Unbundle By Name(w132) -> ("channels"=w131:T2[])
        n46 = Index Array(array=w131, index=w130) -> (element=w129:T2)
        n47 = Unbundle By Name(w129) -> ("F8588"=w128:bool)
        n48 = case shown="True" w128 {
          tunnel: w147 -> [w150 w155]
          tunnel: [w148 w154] -> w146
          tunnel: [w149 w153] -> w145
          tunnel: w142 -> [w151 w152]
          frame True {
            n49 = call "F8588A Async Start Digitizing Process.vi"("error in"=w150, "digitizer session"=w151) -> ("error out"=w149:errorcluster, "vi ref out"=w148:refnum<vi>)  [unwired: 8 in]
          }
          frame False, Default {
            n50 = call "3458A Async Start Digitizing Process.vi"("error in"=w155, "digitizer session"=w152) -> ("error out"=w153:errorcluster, "vi ref out"=w154:refnum<vi>)  [unwired: 8 in]
          }
        }
        n51 = Dequeue Element(queue=w144, timeout in ms (-1)=10000, error in (no error)=w145) -> (element=w135:T40, timed out?=w137:bool, error out=w138:errorcluster)  [unwired: 1 out]
        n52 = Unbundle By Name(w135) -> ("sampling?"=w134:bool)
        n53 = Compound Arithmetic op=OR(invert w134, w137, w138) -> (w136:bool)
      }
      n54 = Bundle By Name(cluster=w56, "proc setup.proc refs"=w55) -> (w54:T1)
      n55 = case shown="No Error" w57 {
        selector: w57 -> [w114 w127]
        tunnel: w54 -> [w113 w126]
        tunnel: [w111 w127] -> w53
        tunnel: [w109 w126] -> w52
        tunnel: [w108 _] -> w30
        frame No Error {
          # "this is used to generate\nestimated sampling progress\nstatus because 3458 returns\nfirst data after completed"
          # "At this point all channels should be ready to\ndigitize or alrady digitizing (TIMER clocked mode)"
          n56 = call "3458A Check Needed Aux HW.vi"("digitizer session"=w113) -> ("uses AWG clocking?"=w115:bool)  [unwired: 13 in, 5 out]
          n57 = case shown="True" w115 {
            tunnel: w114 -> [w118 w125]
            tunnel: w113 -> [w119 w122]
            tunnel: [w118 w121] -> w112
            tunnel: [w119 w120] -> w110
            frame False {
              # "do nothing for TIMER clocked modes"
            }
            frame True {
              # "start clocking for AWG clocked modes"
              n58 = Unbundle By Name(w122) -> ("awg unit"=w124:T5)
              n59 = call "AWG Start Pulses.vi"("error in (no error)"=w125, "awg session in"=w124) -> ("error out"=w121:errorcluster, "awg session out"=w123:T5)  [unwired: 8 in]
              n60 = Bundle By Name(cluster=w122, "awg unit"=w123) -> (w120:T1)
            }
          }
          n61 = flat-sequence {
            tunnel: [w117] -> w111
            tunnel: w112 -> [w117]
            tunnel: [w116] -> w108
            frame #0 {
              n62 = Get Date/Time In Seconds() -> (seconds since 1Jan1904=w116:timestamp)
            }
          }
          n63 = Bundle By Name(cluster=w110, "init timestamp"=w108, "last report timestamp"=w108) -> (w109:T1)
        }
        frame Error {
        }
      }
    }
  }
  "error out" <- w11
  "session out" <- w10
  "initiation timestamp" <- w7
